vi "VarexLib Validate.vi"(11 "AD Group In":string) -> (1 "User ID Out":string, 3 "OK?":bool)   [LabVIEW 2024]
uses:
  C:/Users/bjames/Documents/GitHub/LVAutomation/Support Files/VarexLib.dll
  Support Files/VarexLib.dll
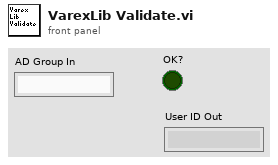
[diagram p1: front panel]
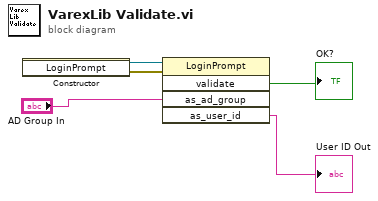
[diagram p0: block diagram]
diagram:
  n1 = constructor class="LoginPrompt"() -> (reference out=w5:refnum<k24>, error out=w4:errorcluster)  [unwired: 3 in, 1 out]
  n2 = invoke class="LoginPrompt" method="validate"(reference=w5, error in=w4, "as_ad_group"="AD Group In") -> ("validate"=→"OK?":bool, "as_user_id"=→"User ID Out":string)  [unwired: 2 in, 3 out]
